vi "finalize initialization.vi"(8 "error in":errorcluster, 10 "configuration in":refnum<class "fixed channel configuration.lvclass">, 11 "Watchdog runtime in":refnum<class "Watchdog runtime.lvclass">) -> (0 "error out":errorcluster, 3 "Watchdog runtime out":refnum<class "Watchdog runtime.lvclass">)   [LabVIEW 2013, in "Watchdog runtime.lvclass"]
uses:
  Watchdog runtime.lvclass
  <vilib>/NI/Tag Bus Data Framework/fixed module parent/module/configuration/fixed channel configuration.lvclass
  configuration/Watchdog configuration.lvclass
  <vilib>/RTwatchdog.llb/Watchdog expiration actions.ctl
  Watchdog runtime.lvclass/Watchdog runtime.ctl
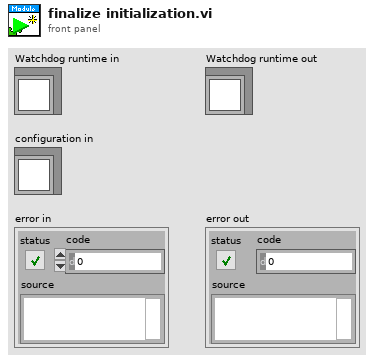
[diagram p1: front panel]
types:
  T1 = typedef "Watchdog expiration actions.ctl" = cluster{"reset":bool, "occurrence":bool, "trigger protocol":enum16{"active high", "active low", "open collector"}, "trigger line":enum16{"none", "line 0", "line 1", "line 2", "line 3", "line 4", "line 5", "line 6", "line 7", "SMB line 0"}, "disable watchdog on VI exit":bool}
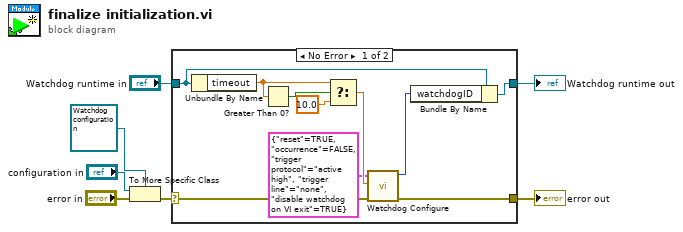
[diagram p0: block diagram]
diagram:
  n1 = To More Specific Class(target class=refnum<class "Watchdog configuration.lvclass"> refnum ("user module configuration"), reference="configuration in", error in="error in") -> (error out=w4:errorcluster)  [unwired: 1 out]
  n2 = case shown="No Error" w4 {
    selector: w4 -> [w13 w18]
    tunnel: [w10 w19] -> w3
    tunnel: "Watchdog runtime in" -> [w17 w19]
    tunnel: [w12 w18] -> w1
    frame No Error {
      n3 = Unbundle By Name(w17) -> ("timeout"=w15:dbl)
      n4 = Greater Than 0?(x=w15) -> (x > 0?=w16:bool)
      n5 = Select(t=w15, s=w16, f=10.0) -> (s? t:f=w11:dbl)
      n6 = call <vilib>:"Watchdog Configure.vi"("error in (no error)"=w13, "expiration actions"=T1 {"reset"=TRUE, "occurrence"=FALSE, "trigger protocol"=enum."active high", "trigger line"=enum."none", "disable watchdog on VI exit"=TRUE}, "timeout (1 sec)"=w11) -> ("error out"=w12:errorcluster, "watchdogID"=w9:u32)  [unwired: 1 in, 2 out]
      n7 = Bundle By Name(cluster=w17, "watchdogID"=w9) -> (w10:refnum<class "Watchdog runtime.lvclass">)
    }
    frame Error {
    }
  }
  "error out" <- w1
  "Watchdog runtime out" <- w3
